vi "PH_Sound.Device Play Tone.vi"(3 "error in":errorcluster, 4 "Length [ms]":u32, 5 "tone":T1 items=["c"=130.8, "cis"=138.6, "d"=146.8, "es"=155.6, "e"=164.8, "f"=174.6, "fis"=185.0, "g"=196.0, "as"=207.6, "a"=220.0, "b"=233.1, "h"=246.9, "c'"=261.6, "cis'"=277.2, "d'"=293.7, "es'"=311.1, "e'"=329.6, "f'"=349.2, "fis'"=370.0, "g'"=392.0, "as'"=415.3, "a'"=440.0, "b'"=466.2, "h'"=493.9, "c''"=523.3, "cis''"=554.4, "d''"=587.3, "es''"=622.3, "e''"=659.3, "f''"=689.5, "fis''"=740.0, "g''"=784.0, "as''"=830.6, "a''"=880.0, "b''"=932.3, "h''"=987.8, "c'''"=1047.0]) -> (0 "Device error out":errorcluster)   [LabVIEW 2014, in "PH_Sound.lvlib"]
uses:
  PH_Sound.lvlib
  PH_Sound.3Oktaves.ctl
  <vilib>/sound2/lvsound2.llb/Sound Data Format.ctl
  <vilib>/sound2/lvsound2.llb/Sampling Mode.ctl
  <vilib>/sound2/lvsound2.llb/Sound Output Write (DBL Single).vi
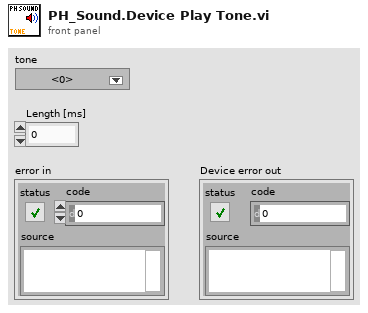
[diagram p1: front panel]
types:
  T1 = typedef "PH_Sound.lvlib/PH_Sound.3Oktaves.ctl" = dbl
  T2 = typedef "Sampling Mode.ctl" = i32
  T3 = typedef "Sound Data Format.ctl" = cluster{"sample rate (S/s)":dbl, "number of channels":i32, "bits per sample":i32}
  T4 = typedef "Sound Output Task ID.ctl" = u32
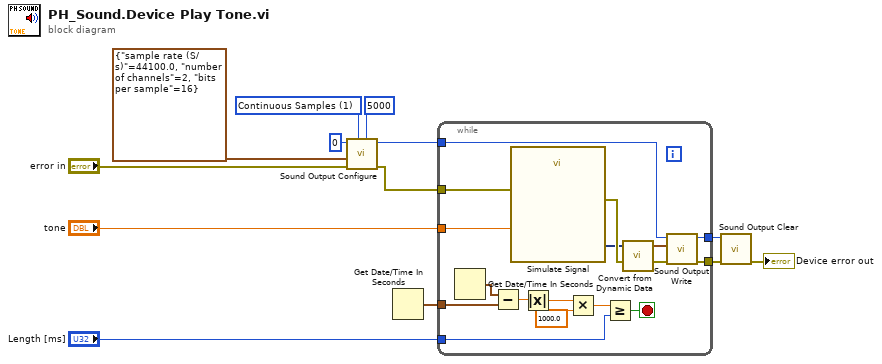
[diagram p0: block diagram]
diagram:
  w6 = T2 1 items=["Finite Samples", "Continuous Samples"] ("sample mode")
  n1 = call <vilib>:"Sound Output Configure.vi"("number of samples/ch"=5000, "sample mode"=w6, "error in (no error)"="error in", "sound format"=T3 {"sample rate (S/s)"=44100.0, "number of channels"=2, "bits per sample"=16}, "device ID"=u32 0) -> ("error out"=w3:errorcluster, "task ID"=w1:T4)  [unwired: 5 in]
  n2 = Get Date/Time In Seconds() -> (seconds since 1Jan1904=w12:timestamp)
  n3 = while {
    tunnel: w1 -> [w28]
    tunnel: "tone" -> [w15]
    tunnel: w12 -> [w23]
    tunnel: "Length [ms]" -> [w18]
    tunnel: w3 -> [w29]
    tunnel: [w17] -> w9
    tunnel: [w14] -> w8
    stop <- w16 stop-if-true
    n4 = Get Date/Time In Seconds() -> (seconds since 1Jan1904=w24:timestamp)
    n5 = Subtract(x=w24, y=w23) -> (x-y=w22:dbl)
    n6 = call "Simulate Signal"("Frequency"=w15, "error in (no error)"=w29) -> ("Sine"=w26:dynamicdata, "error out"=w27:errorcluster)  [unwired: 12 in]
    n7 = Absolute Value(x=w22) -> (abs(x)=w21:dbl)
    n8 = Multiply(x=w21, y=1000.0) -> (x*y=w19:dbl)
    n9 = Greater Or Equal?(x=w19, y=w18) -> (x >= y?=w16:bool)
    n10 = call "Convert from Dynamic Data"("Dynamic Data Type"=w26) -> ("Waveform"=w25:waveform(dbl))  [unwired: 3 in]
    n11 = call-poly <vilib>:"Sound Output Write.vi"("error in (no error)"=w27, "data"=w25, "task ID"=w28) -> ("error out"=w17:errorcluster, "task ID out"=w14:T4)  [unwired: 7 in]
  }
  n12 = call <vilib>:"Sound Output Clear.vi"("error in (no error)"=w9, "task ID"=w8) -> ("error out"=→"Device error out":errorcluster)  [unwired: 9 in]
